vi "Read Start Point.vi"(2 "error in (no error)":errorcluster, 3 "Line.lvclass":refnum<class "Line.lvclass">) -> (0 "error out":errorcluster, 1 "Start Point.lvclass":refnum<class "Point.lvclass">)   [LabVIEW 2015, in "Line.lvclass"]
uses:
  Line.lvclass
  Point.lvclass
  Line.lvclass/Line.ctl
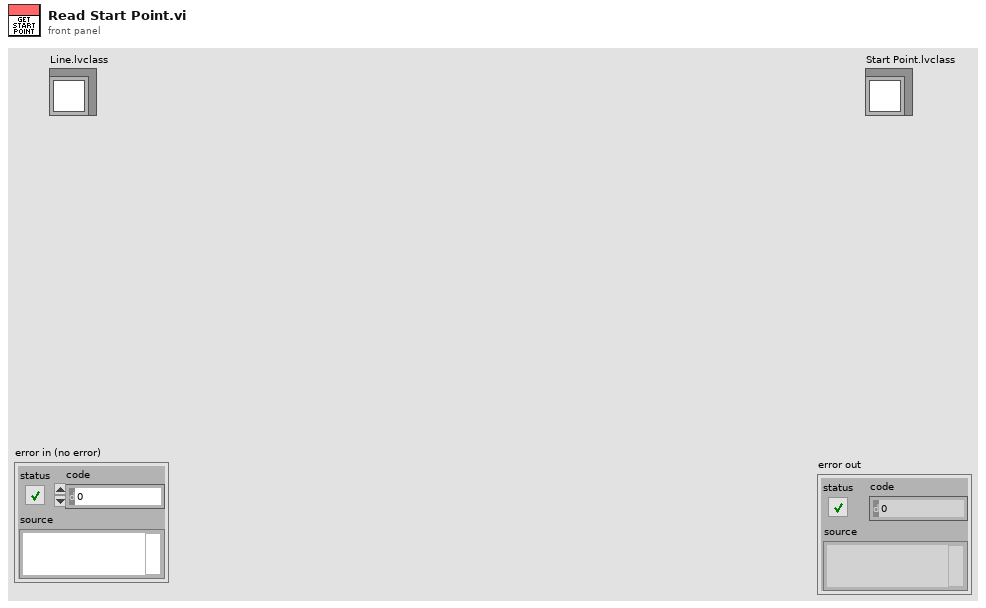
[diagram p1: front panel]
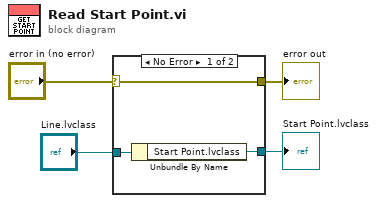
[diagram p0: block diagram]
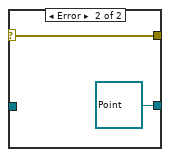
[diagram p2: hidden frame]
diagram:
  n1 = case shown="No Error" "error in (no error)" {
    selector: "error in (no error)" -> [w7 w9]
    tunnel: [w7 w9] -> w3
    tunnel: "Line.lvclass" -> [w6 _]
    tunnel: [w5 refnum<class "Point.lvclass"> refnum ("Point.lvclass")] -> w1
    frame No Error {
      n2 = Unbundle By Name(w6) -> ("Start Point.lvclass"=w5:refnum<class "Point.lvclass">)
    }
    frame Error {
    }
  }
  "error out" <- w3
  "Start Point.lvclass" <- w1
